vi "URExample.vi"() -> ()   [LabVIEW 2014]
uses:
  Z:/UnderAutomationDev/Submodules/Samples/Libraries/net35/UnderAutomation.UniversalRobots.dll
  Libraries/net35/UnderAutomation.UniversalRobots.dll
panel:
  in  "GetPose() Answer":T1={"X"=1.0, "Y"=-2.1, "Z"=1.0, "RX"=0.1, "RY"=-0.1, "RZ"=0.0}
  out "Method":string
  in  "Default Answer":string="Hello Robot !"
  out "IP PC :":string
  in  "URScript":string
  out "Command error":errorcluster
  in  "Execute script":bool
  in  "Realease brake":bool
  in  "Power On":bool
  out "Z":dbl
  out "Y":dbl
  out "DataError":errorcluster caption="error out 2"
  out "X":dbl
  out "LicenseInfo":string
  out "Connect Error":errorcluster
  in  "ip":string="192.168.0.56"
  in  "Connect":bool
  out "Connected":bool
  out "error out":errorcluster
  # "Read data"
  # "Connect"
  # "XML RPC"
  # "Use this code on your robot to ask LabView some data (change the IP with IP of this machine)\n\nrpc:=rpc_factory(\"xmlrpc\", \"http://192.168.0.1:50000\")\nanswer:=rpc.GetPose()"
  # "Last method called by the robot :"
  # "Answer (String) returned else :"
  # "Answer (Pose) returned when\nmethod \"GetPose\" is called :"
  # "Send commands"
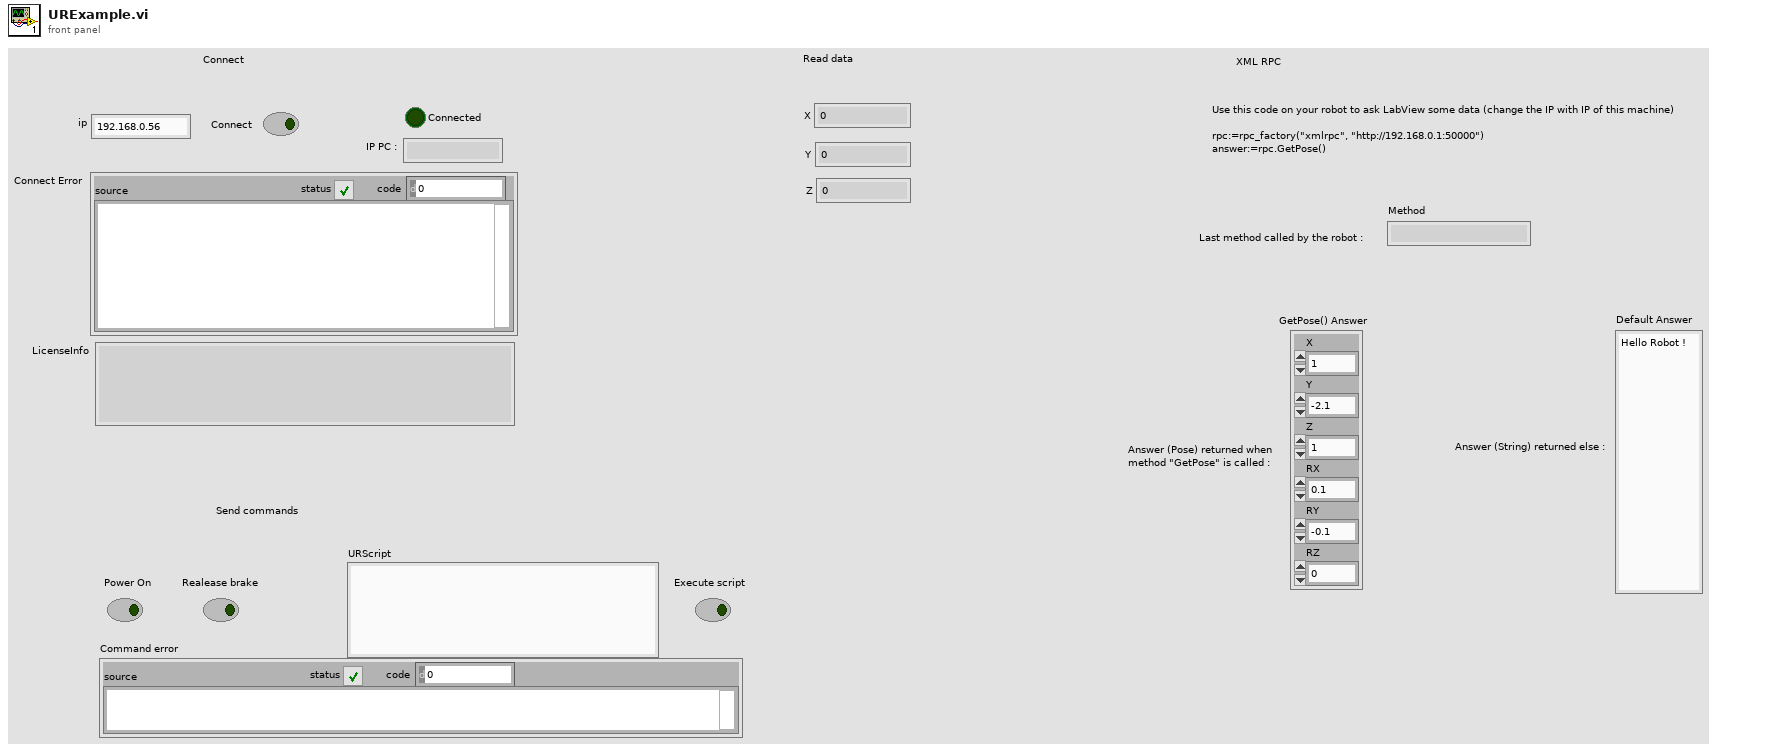
[diagram p1: front panel]
types:
  T1 = cluster{"X":dbl, "Y":dbl, "Z":dbl, "RX":dbl, "RY":dbl, "RZ":dbl}
  T2 = cluster{"Method":refnum<vi>, "Default Answer":refnum<vi>, "GetPose() Answer":cluster{"X":dbl, "Y":dbl, "Z":dbl, "RX":dbl, "RY":dbl, "RZ":dbl}}
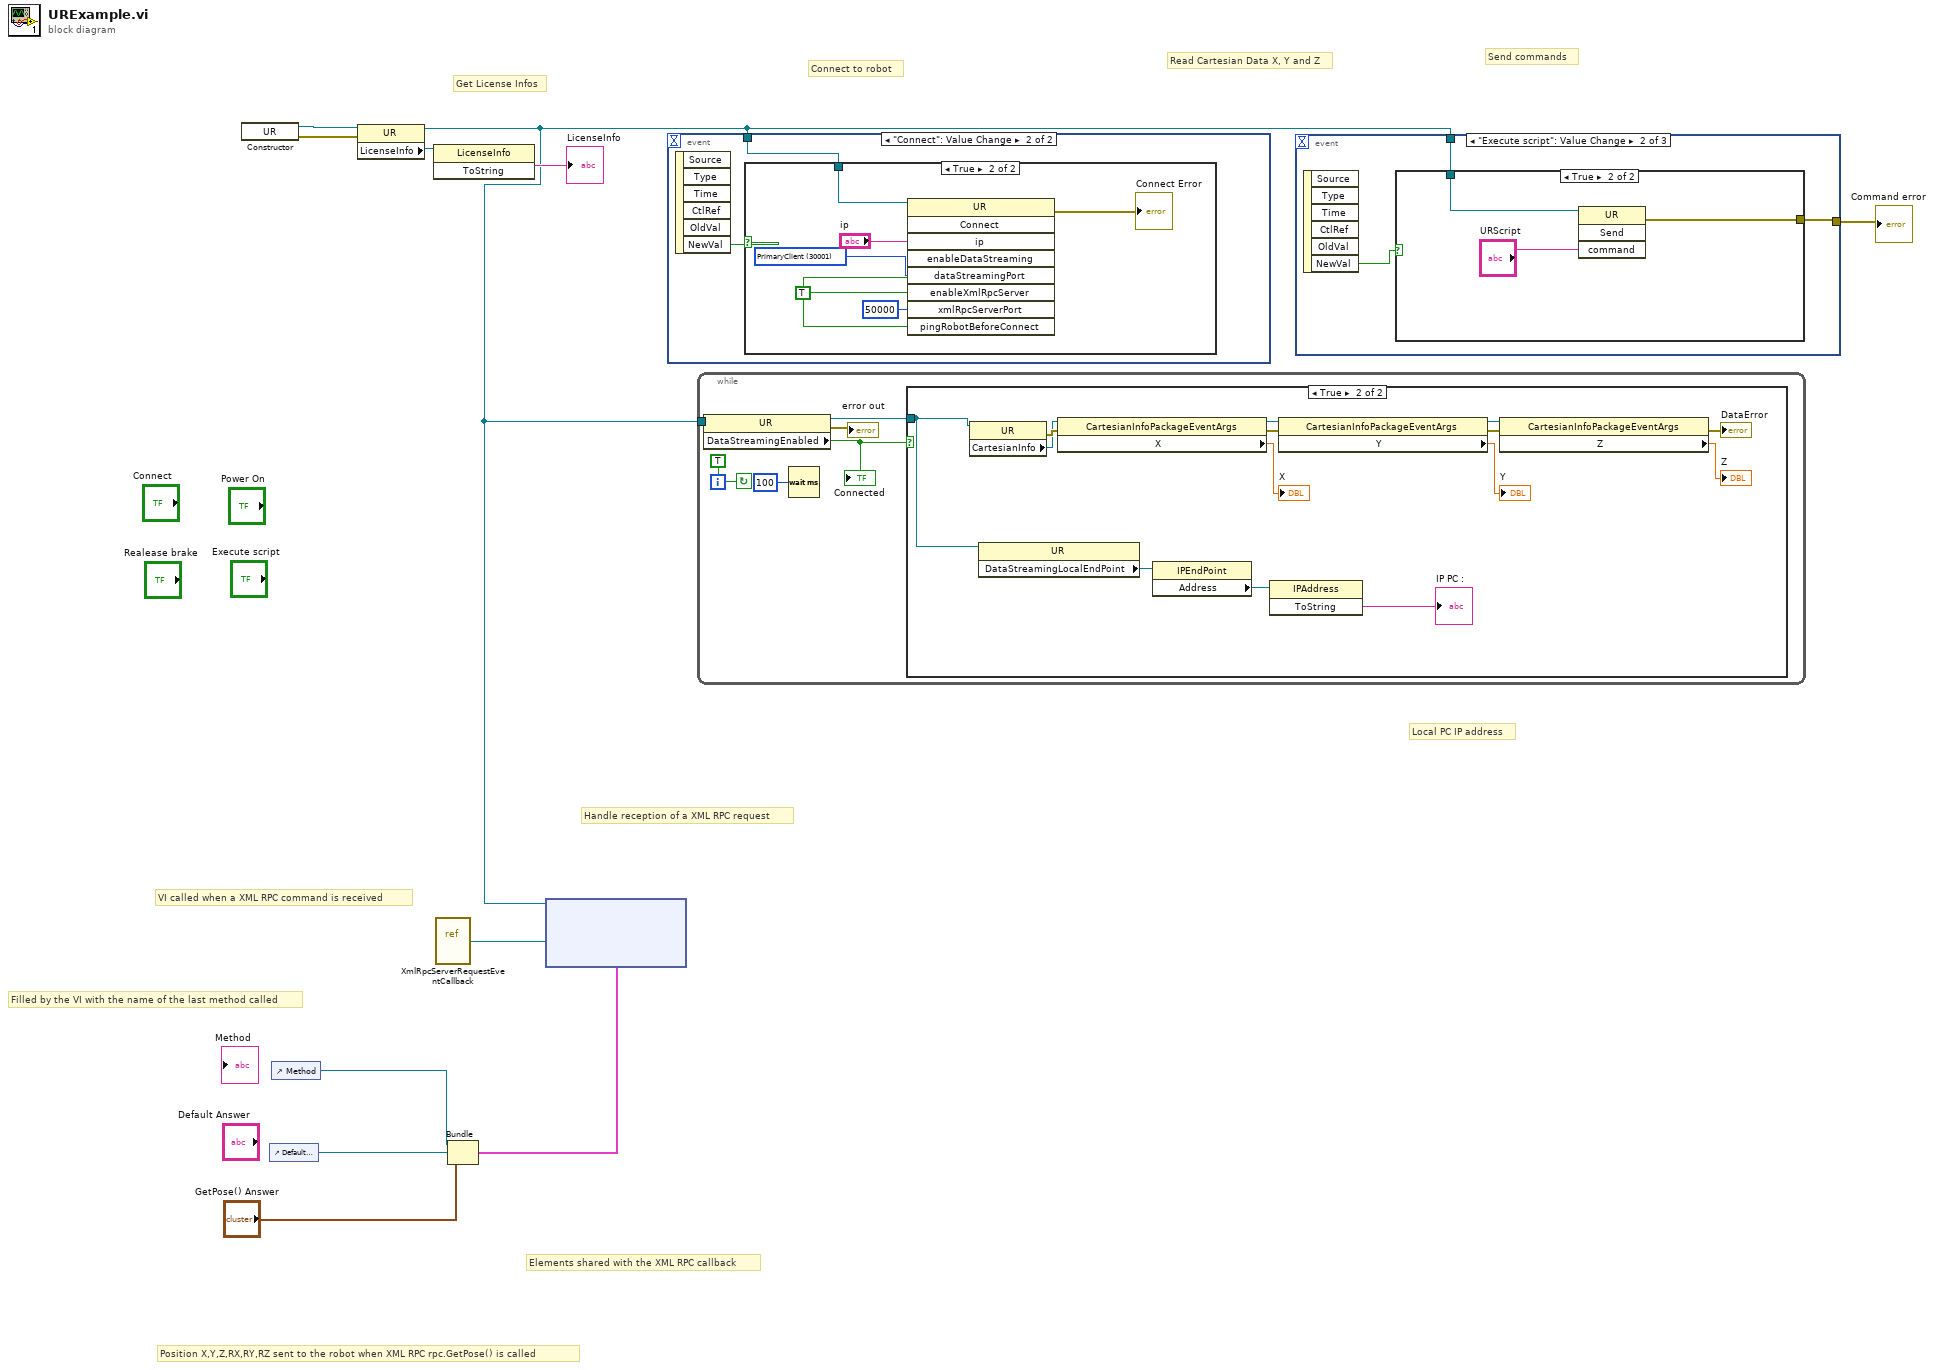
[diagram p0: block diagram]
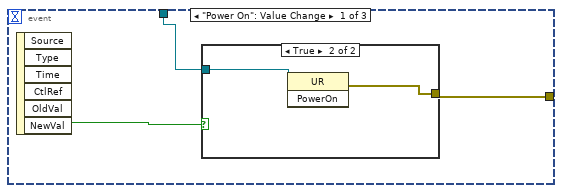
[diagram p2: hidden frame]
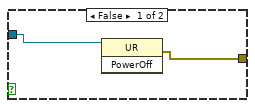
[diagram p3: hidden frame]
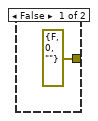
[diagram p4: hidden frame]
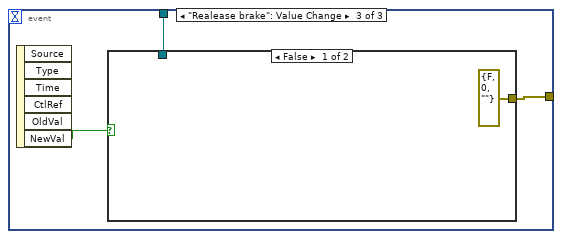
[diagram p5: hidden frame]
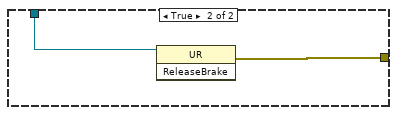
[diagram p6: hidden frame]
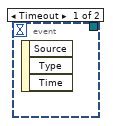
[diagram p7: hidden frame]
diagram:
  # "Filled by the VI with the name of the last method called"
  # "Position X,Y,Z,RX,RY,RZ sent to the robot when XML RPC rpc.GetPose() is called"
  # "Elements shared with the XML RPC callback"
  # "VI called when a XML RPC command is received"
  # "Handle reception of a XML RPC request"
  # "Local PC IP address"
  # "Send commands"
  # "Connect to robot"
  # "Get License Infos"
  # "Read Cartesian Data X, Y and Z"
  n1 = constructor class="UR"() -> (reference out=w7:refnum<k24>, error out=w11:errorcluster)  [unwired: 3 in, 1 out]
  n2 = control-ref of="Default Answer"() -> (w5:refnum<vi>)
  n3 = control-ref of="Method"() -> (w6:refnum<vi>)
  n4 = property class="UR"(reference=w7, error in=w11) -> (reference out=w3:refnum<k24>, "LicenseInfo"=w10:refnum<k24>)  [unwired: 1 out]
  n5 = invoke class="LicenseInfo" method="ToString"(reference=w10) -> ("ToString"=→"LicenseInfo":string)  [unwired: 2 in, 2 out]
  n6 = vi-ref "XmlRpcServerRequestEventCallback.vi"() -> ("vi reference"=w2:refnum<vi>)
  n7 = Bundle("Method"=w6, "Default Answer"=w5, "GetPose() Answer"="GetPose() Answer") -> (w4:T2)  [unwired: 1 in]
  n8 = node(w3, w2, w4) -> ()  [unwired: 2 in, 2 out]
  n9 = event shown="[1] \"Connect\": Value Change" {
    selector: _ -> [_ _]
    dyn-events: _ -> [_ _]
    timeout: _ -> [_ _]
    tunnel: w3 -> [_ w12]
    event Timeout {
      n10 = event-data() -> ()  [unwired: 1 in, 3 out]
    }
    event "Connect": Value Change {
      n11 = event-data() -> ("NewVal"=w13:bool)  [unwired: 1 in, 5 out]
      n12 = case shown="True" w13 {
        tunnel: w12 -> [_ w18]
        frame False {
        }
        frame True {
          w15 = TRUE ("listenStreamingInterface")
          w17 = 30001 items=["PrimaryClient"=30001, "SecondaryClient"=30002, "PrimaryClientReadOnly"=30011, "SecondaryClientReadOnly"=30012] ("port")
          n13 = invoke class="UR" method="Connect"(reference=w18, "ip"="ip", "enableDataStreaming"=w15, "dataStreamingPort"=w17, "enableXmlRpcServer"=w15, "xmlRpcServerPort"=50000, "pingRobotBeforeConnect"=w15) -> (error out=→"Connect Error":errorcluster)  [unwired: 2 in, 8 out]
        }
      }
    }
  }
  n14 = while {
    tunnel: w3 -> [w23]
    stop <- TRUE continue-if-true
    n15 = property class="UR"(reference=w23) -> (reference out=w20:refnum<k24>, error out=→"error out":errorcluster, "DataStreamingEnabled"=w22:bool)  [unwired: 1 in]
    "Connected" <- w22
    n16 = Wait (ms)(milliseconds to wait=u32 100) -> ()  [unwired: 1 out]
    n17 = case shown="True" w22 {
      tunnel: w20 -> [_ w26]
      frame False {
      }
      frame True {
        n18 = property class="UR"(reference=w26) -> (error out=w32:errorcluster, "CartesianInfo"=w30:refnum<k24>)  [unwired: 1 in, 1 out]
        n19 = property class="UR"(reference=w26) -> ("DataStreamingLocalEndPoint"=w27:refnum<k24>)  [unwired: 1 in, 2 out]
        n20 = property class="CartesianInfoPackageEventArgs"(reference=w30, error in=w32) -> (reference out=w35:refnum<k24>, error out=w36:errorcluster, "X"=→"X":dbl)
        n21 = property class="IPEndPoint"(reference=w27) -> ("Address"=w28:refnum<k24>)  [unwired: 1 in, 2 out]
        n22 = invoke class="IPAddress" method="ToString"(reference=w28) -> ("ToString"=→"IP PC :":string)  [unwired: 2 in, 2 out]
        n23 = property class="CartesianInfoPackageEventArgs"(reference=w35, error in=w36) -> (reference out=w33:refnum<k24>, error out=w34:errorcluster, "Y"=→"Y":dbl)
        n24 = property class="CartesianInfoPackageEventArgs"(reference=w33, error in=w34) -> (error out=→"DataError":errorcluster, "Z"=→"Z":dbl)  [unwired: 1 out]
      }
    }
  }
  n25 = event shown="[1] \"Execute script\": Value Change" {
    selector: _ -> [_ _ _]
    dyn-events: _ -> [_ _ _]
    timeout: _ -> [_ _ _]
    tunnel: w3 -> [w41 w49 w56]
    tunnel: [w40 w48 w54] -> w8
    event "Power On": Value Change {
      n26 = event-data() -> ("NewVal"=w42:bool)  [unwired: 1 in, 5 out]
      n27 = case shown="True" w42 {
        tunnel: [w43 w46] -> w40
        tunnel: w41 -> [w44 w45]
        frame False {
          n28 = invoke class="UR" method="PowerOff"(reference=w44) -> (error out=w43:errorcluster)  [unwired: 2 in, 2 out]
        }
        frame True {
          n29 = invoke class="UR" method="PowerOn"(reference=w45) -> (error out=w46:errorcluster)  [unwired: 2 in, 2 out]
        }
      }
    }
    event "Execute script": Value Change {
      n30 = event-data() -> ("NewVal"=w47:bool)  [unwired: 1 in, 5 out]
      n31 = case shown="True" w47 {
        tunnel: w49 -> [_ w53]
        tunnel: [errorcluster {"status"=FALSE, "code"=0, "source"=""} ("error out") w52] -> w48
        frame False {
        }
        frame True {
          n32 = invoke class="UR" method="Send"(reference=w53, "command"="URScript") -> (error out=w52:errorcluster)  [unwired: 2 in, 3 out]
        }
      }
    }
    event "Realease brake": Value Change {
      n33 = event-data() -> ("NewVal"=w55:bool)  [unwired: 1 in, 5 out]
      n34 = case shown="False" w55 {
        tunnel: w56 -> [_ w59]
        tunnel: [errorcluster {"status"=FALSE, "code"=0, "source"=""} ("error out") w58] -> w54
        frame False {
        }
        frame True {
          n35 = invoke class="UR" method="ReleaseBrake"(reference=w59) -> (error out=w58:errorcluster)  [unwired: 2 in, 2 out]
        }
      }
    }
  }
  "Command error" <- w8
